vi "MRU_SP (SubVI).vi"(0 "MT_DATA":sgl[](array[numeric])=[0.0, 0.0, 0.0, 0.0, 0.0, 0.0, 0.0, 0.0, 0.0, 0.0, 0.0, 0.0], 1 "Reset MRU heading":bool, 2 "w/ reset heading":bool, 5 "psi select":u16(ring) items=["Compass heading", "MRU heading", "MTI heading"], 7 "Signals out in":dbl[](array[numeric]), 9 "MRU out":dbl[](array[numeric]), 13 "Reset MTI heading":bool) -> (3 "MRU psi mod":dbl, 4 "MRU r":dbl, 6 "MRU psi":dbl, 10 "w":dbl, 12 "Signals out out":dbl[](array[numeric]), 14 "r":dbl, 15 "psi off":dbl)   [LabVIEW 2011]
uses:
  <vilib>/imath/engines/lvmath2/RunTimeEngine/ErrorHandling/NIMS_Finalize Error.vi
  <vilib>/imath/engines/lvmath2/RunTimeEngine/NodeEndStatement/NIMS_NodeEndStatement_Get Vector.vi
  <instcachedir>/0/NIMS_NodeEndStatement_Get Vector_50E2F48DC826428EA11CD85545CBACBE.lvgen/NIMS_NodeEndStatement_Get Vector_50E2F48DC826428EA11CD85545CBACBE_001.vi
  <vilib>/imath/engines/lvmath2/RunTimeEngine/NodeEndStatement/NIMS_NodeEndStatement_Output.vi
  <instcachedir>/0/NIMS_NodeEndStatement_Output_53EC0D466D134D7ABD903AC30B43404B.lvgen/NIMS_NodeEndStatement_Output_53EC0D466D134D7ABD903AC30B43404B_005.vi
  <vilib>/imath/engines/lvmath2/RunTimeEngine/ArithmeticOperatorToken/NIMS_ArithmeticOperator_multmx(M,CV).vi
  <instcachedir>/0/NIMS_ArithmeticOperator_multmx(M,CV)_B95E4EDD04E247939487CF1FF34819AA.lvgen/NIMS_ArithmeticOperator_multmx(M,CV)_B95E4EDD04E247939487CF1FF34819AA_007.vi
  <vilib>/imathl/engines/lvmath/Functions/Error Handling/Create Error.vi
panel:
  out "psi off 2":dbl
  out "acc_t":dbl[](array[numeric])
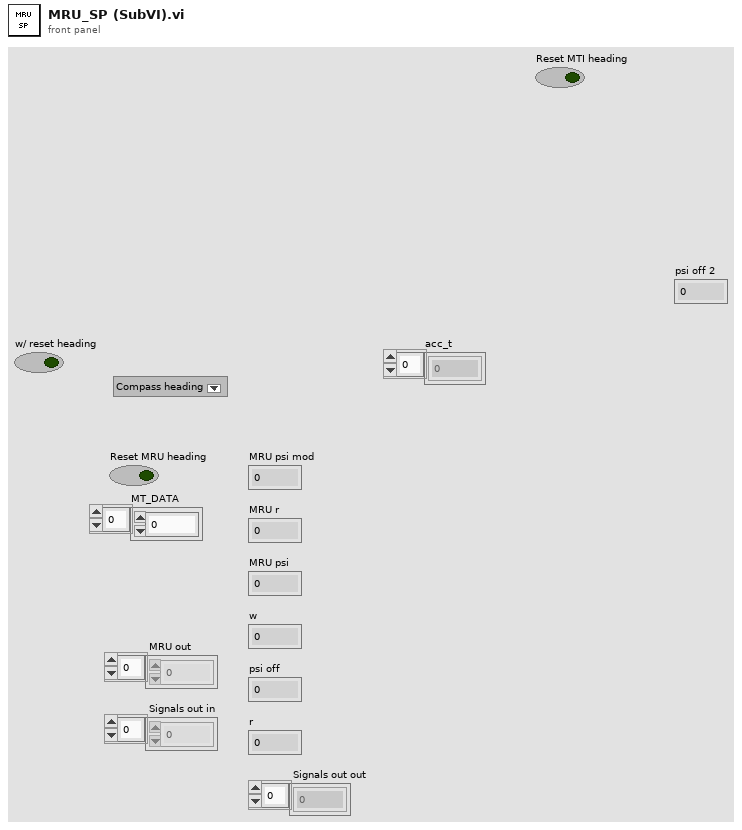
[diagram p1: front panel]
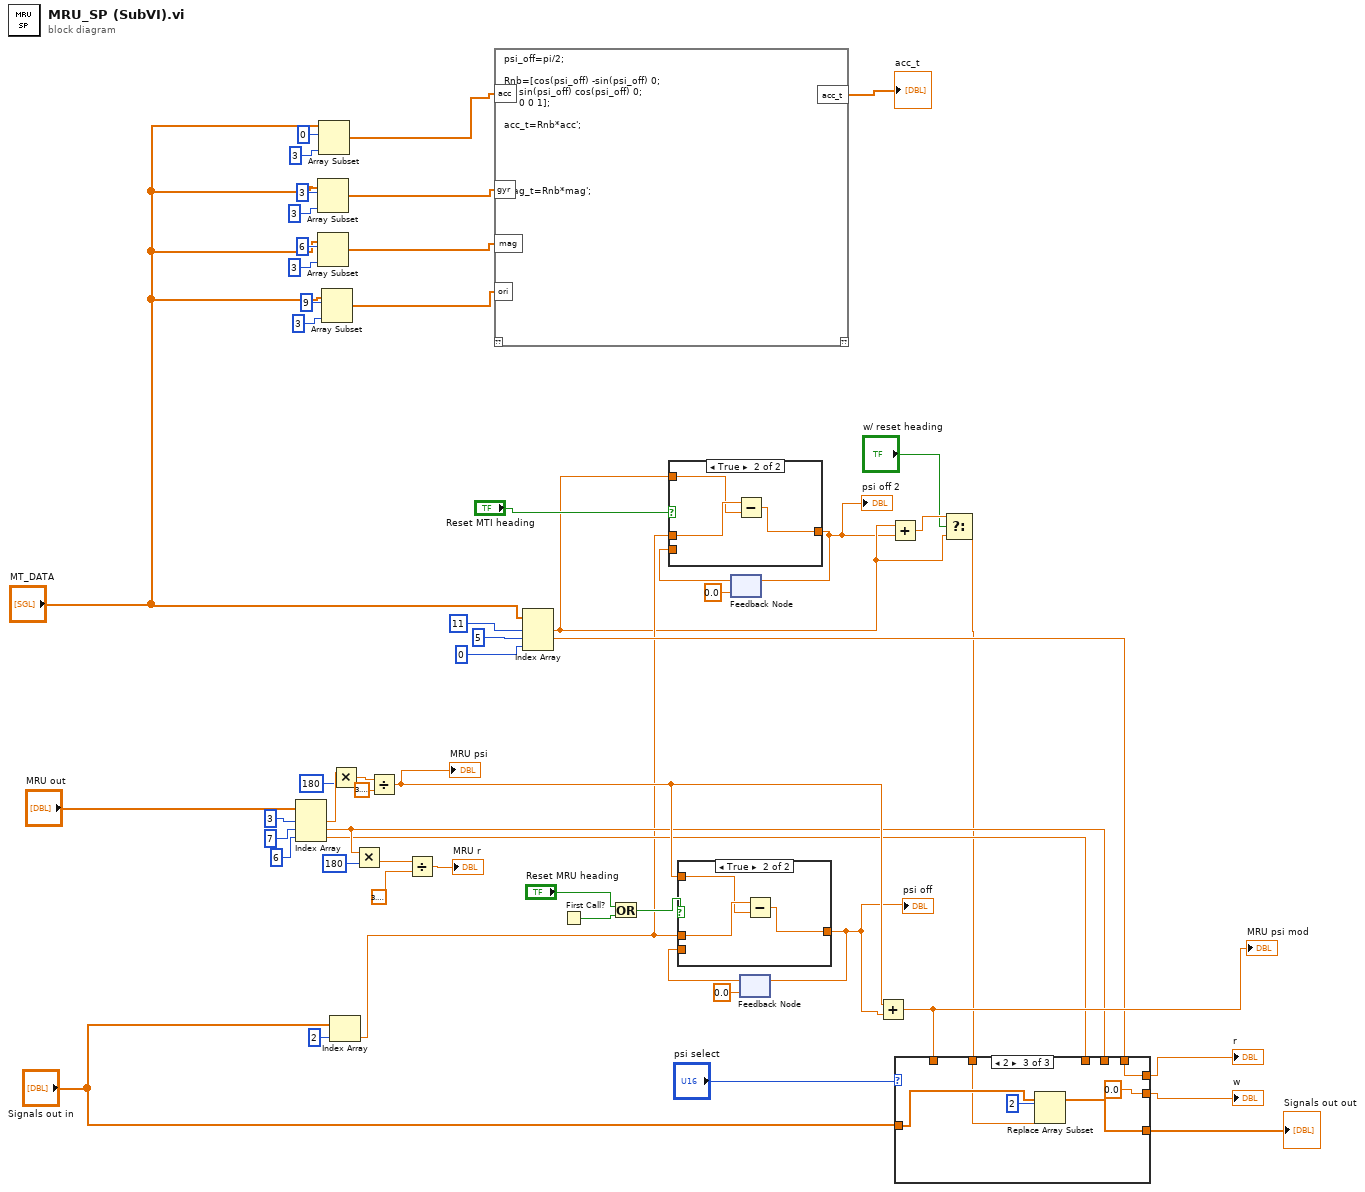
[diagram p0: block diagram]
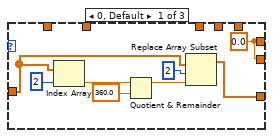
[diagram p4: hidden frame]
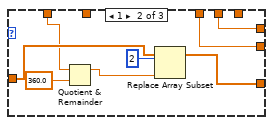
[diagram p5: hidden frame]
diagram:
  n1 = Index Array(array="MRU out", index #1=3 ("index"), index #2=7 ("index"), index #3=6 ("index")) -> (element #1=w41:dbl, element #2=w31:dbl, element #3=w29:dbl)
  n2 = Array Subset(array="MT_DATA", index=3, length=3) -> (w14:sgl[])
  n3 = Array Subset(array="MT_DATA", index=6, length=3) -> (w13:sgl[])
  n4 = Array Subset(array="MT_DATA", index=0, length=3) -> (w22:sgl[])
  n5 = Array Subset(array="MT_DATA", index=9, length=3) -> (w12:sgl[])
  n6 = Index Array(array="Signals out in", index=2) -> (element=w8:dbl)
  n7 = Multiply(x=w41, y=180 ("index")) -> (x*y=w38:dbl)
  n8 = Multiply(x=w31, y=180 ("index")) -> (x*y=w45:dbl)
  n9 = Divide(x=w38, y=3.141592653589793) -> (x/y=w51:dbl)
  "MRU psi" <- w51
  n10 = Divide(x=w45, y=3.141592653589793) -> (x/y=→"MRU r":dbl)
  n11 = mathscript code="psi_off=pi/2;\n\nRnb=[cos(psi_off) -sin(psi_off) 0;\n     sin(psi_off) cos(psi_off) 0;\n     0 0 1];\n\nacc_t=Rnb*acc';\n\n\n\n\n\nmag_t=Rnb*mag';"("acc"=w22, "gyr"=w14, "mag"=w13, "ori"=w12) -> ("acc_t"=→"acc_t":dbl[])  [unwired: 1 in, 1 out]
  n12 = Index Array(array="MT_DATA", index #1=11 ("index"), index #2=5 ("index"), index #3=0 ("index")) -> (element #1=w6:sgl, element #2=w26:sgl)  [unwired: 1 out]
  n13 = First Call?() -> (First Call?: T/F=w48:bool)
  n14 = Or(x="Reset MRU heading", y=w48) -> (x .or. y?=w50:bool)
  n15 = feedback #1(0.0) -> (w9:dbl)
  n16 = case shown="True" "Reset MTI heading" {
    tunnel: w8 -> [_ w59]
    tunnel: w6 -> [_ w58]
    tunnel: [w56 w57] -> w1
    tunnel: w9 -> [w56 _]
    frame False {
    }
    frame True {
      n17 = Subtract(x=w59, y=w58) -> (x-y=w57:dbl)
    }
  }
  "psi off 2" <- w1
  n18 = feedback-in #1(w1) -> ()
  n19 = feedback #2(0.0) -> (w35:dbl)
  n20 = case shown="True" w50 {
    tunnel: w8 -> [_ w63]
    tunnel: w51 -> [_ w62]
    tunnel: [w60 w61] -> w2
    tunnel: w35 -> [w60 _]
    frame False {
    }
    frame True {
      n21 = Subtract(x=w63, y=w62) -> (x-y=w61:dbl)
    }
  }
  "psi off" <- w2
  n22 = feedback-in #2(w2) -> ()
  n23 = Add(x=w51, y=w2) -> (x+y=w52:dbl)
  "MRU psi mod" <- w52
  n24 = Add(x=w6, y=w1) -> (x+y=w5:dbl)
  n25 = Select(t=w5, s="w/ reset heading", f=w6) -> (s? t:f=w4:dbl)
  n26 = case shown="2" "psi select" {
    tunnel: "Signals out in" -> [w66 w79 w84]
    tunnel: w52 -> [_ w75 _]
    tunnel: [w65 w77 w82] -> w42
    tunnel: w4 -> [_ _ w83]
    tunnel: w31 -> [_ w73 _]
    tunnel: [w64 w73 w81] -> w30
    tunnel: w29 -> [_ w72 _]
    tunnel: [w64 w72 0.0] -> w28
    tunnel: w26 -> [_ _ w81]
    frame 0, Default {
      w64 = 0.0
      n27 = Index Array(array=w66, index=2) -> (element=w67:dbl)
      n28 = Quotient & Remainder(x=w67, y=360.0) -> (x-y*floor(x/y)=w69:dbl)  [unwired: 1 out]
      n29 = Replace Array Subset(array=w66, new element=w69, index=2) -> (w65:dbl[])
    }
    frame 1 {
      n30 = Quotient & Remainder(x=w75, y=360.0) -> (x-y*floor(x/y)=w74:dbl)  [unwired: 1 out]
      n31 = Replace Array Subset(array=w79, new element=w74, index=2) -> (w77:dbl[])
    }
    frame 2 {
      n32 = Replace Array Subset(array=w84, new element=w83, index=2) -> (w82:dbl[])
    }
  }
  "w" <- w28
  "r" <- w30
  "Signals out out" <- w42
